vi "波形采集.vi"(2 "rate":dbl=4000.0, 3 "number of samples":i32=1000, 5 "error in":errorcluster) -> ()   [LabVIEW 2010]
doc: "Creates, edits, and runs tasks using NI-DAQmx. Refer to the DAQ Quick Start Guide for information on devices supported by NI-DAQmx.\n\nWhen you place this Express VI on the block diagram, the DAQ Assistant launches to create a new task. After you create a task, you can double-click the DAQ Assistant Express VI in order to edit that task. For continuous measurement or generation, place a loop around the DAQ Assistant Express VI. \n\nFor continuous single-point input or output, the DAQ Assistant Express VI might not provide satisfactory performance. Refer to examples\\DAQmx\\Analog In\\Measure Voltage.llb\\Cont Acq&Graph Voltage-Single Point Optimization.vi for techniques to create higher-performance, single-point I/O applications."
uses:
  <vilib>/DAQmx/read.llb/DAQmx Read (Analog 1D Wfm NChan NSamp).vi
  <vilib>/DAQmx/configure/timing.llb/DAQmx Timing (Sample Clock).vi
  <vilib>/DAQmx/create/channels.llb/DAQmx Create Channel (TEDS-AI-Voltage-Basic).vi
  <vilib>/DAQmx/create/channels.llb/DAQmx Create Channel (AI-Voltage-Basic).vi
  <vilib>/daqmx/miscellaneous.llb/DAQmx Fill In Error Info.vi
panel:
  in  "停止":bool
  out "波形图":waveform(dbl)[](graph)
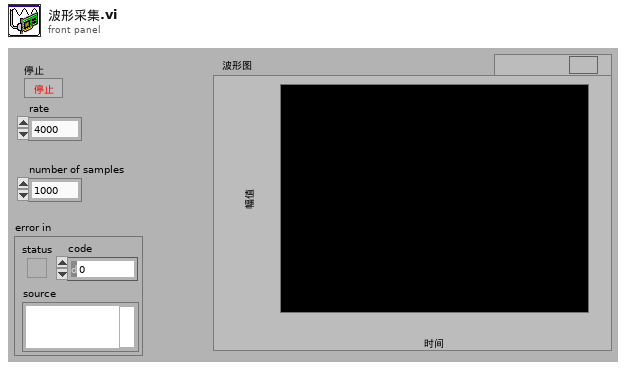
[diagram p1: front panel]
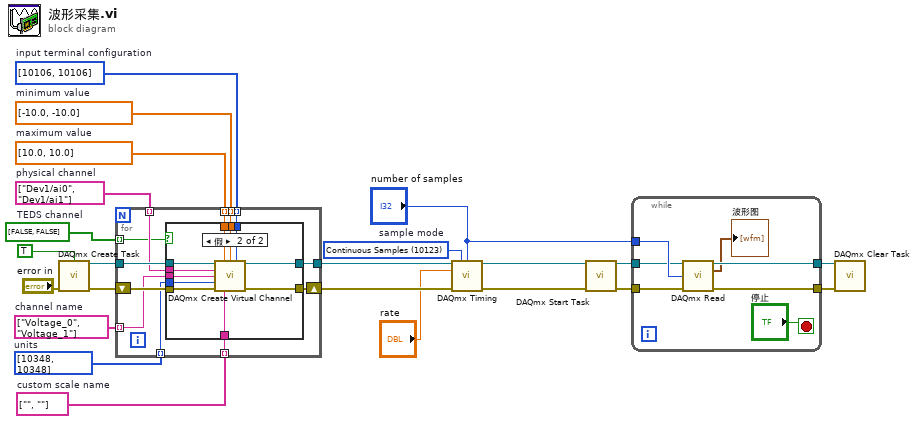
[diagram p0: block diagram]
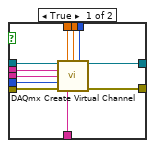
[diagram p2: hidden frame]
diagram:
  w6 = 10123 items=["Finite Samples"=10178, "Continuous Samples"=10123, "Hardware Timed Single Point"=12522]  # sample mode
  w11 = bool[] [FALSE, FALSE]  # TEDS channel
  w12 = string[] ["", ""]  # custom scale name
  w13 = i32[] [10348, 10348] items=["Volts"=10348, "From TEDS"=12516, "From Custom Scale"=10065]  # units
  w14 = string[] ["Voltage_0", "Voltage_1"]  # channel name
  w15 = string[] ["Dev1/ai0", "Dev1/ai1"]  # physical channel
  w16 = dbl[] [10.0, 10.0]  # maximum value
  w17 = dbl[] [-10.0, -10.0]  # minimum value
  w18 = i32[] [10106, 10106] items=["default"=-1, "RSE"=10083, "NRSE"=10078, "Differential"=10106, "Pseudodifferential"=12529]  # input terminal configuration
  n1 = call <vilib>:"DAQmx Create Task.vi"("auto cleanup"=TRUE, "error in"="error in") -> ("task out"=w23:refnum<k21>, "error out"=w22:errorcluster)  [unwired: 12 in]
  n2 = for "For循环" {
    tunnel: w23 -> [w35]
    tunnel: [w33] -> w20
    tunnel: w18 -> [w31] mode=indexing
    tunnel: w17 -> [w30] mode=indexing
    tunnel: w16 -> [w29] mode=indexing
    tunnel: w15 -> [w28] mode=indexing
    tunnel: w14 -> [w27] mode=indexing
    tunnel: w13 -> [w26] mode=indexing
    tunnel: w12 -> [w25] mode=indexing
    shift-right: [w32] -> w19
    shift-left: w22 -> [w34]
    tunnel: w11 -> [w24] mode=indexing
    n3 = case "条件结构" shown="假" w24 {
      tunnel: w35 -> [w46 w57]
      tunnel: w34 -> [w45 w56]
      tunnel: [w44 w55] -> w33
      tunnel: [w43 w54] -> w32
      tunnel: w31 -> [w42 w53]
      tunnel: w30 -> [w41 w52]
      tunnel: w29 -> [w40 w51]
      tunnel: w28 -> [w39 w50]
      tunnel: w27 -> [w38 w49]
      tunnel: w26 -> [w37 w48]
      tunnel: w25 -> [w36 w47]
      frame True {
        n4 = call-poly <vilib>:"DAQmx Create Virtual Channel.vi"("task in"=w46, "maximum value"=w40, "minimum value"=w41, "input terminal configuration"=w42, "physical channels"=w39, "name to assign"=w38, "units"=w37, "error in"=w45, "custom scale name"=w36) -> ("task out"=w44:refnum<k21>, "error out"=w43:errorcluster)  [unwired: 5 in]
      }
      frame False {
        n5 = call-poly <vilib>:"DAQmx Create Virtual Channel.vi"("task in"=w57, "maximum value"=w51, "minimum value"=w52, "input terminal configuration"=w53, "physical channels"=w50, "name to assign"=w49, "units"=w48, "error in"=w56, "custom scale name"=w47) -> ("task out"=w55:refnum<k21>, "error out"=w54:errorcluster)  [unwired: 5 in]
      }
    }
  }
  n6 = call-poly <vilib>:"DAQmx Timing.vi"("task/channels in"=w20, "sample mode"=w6, "samples per channel"="number of samples", "rate"="rate", "error in"=w19) -> ("task out"=w10:refnum<k21>, "error out"=w9:errorcluster)  [unwired: 9 in]
  n7 = call <vilib>:"DAQmx Start Task.vi"("task/channels in"=w10, "error in"=w9) -> ("task out"=w5:refnum<k21>, "error out"=w4:errorcluster)  [unwired: 12 in]
  n8 = while {
    tunnel: "number of samples" -> [w64]
    tunnel: w5 -> [w63]
    tunnel: w4 -> [w62]
    tunnel: [w61] -> w1
    tunnel: [w60] -> w2
    stop <- "停止" stop-if-true
    n9 = call-poly <vilib>:"DAQmx Read.vi"("task/channels in"=w63, "number of samples per channel"=w64, "error in"=w62) -> ("task out"=w60:refnum<k21>, "data"=→"波形图":waveform(dbl)[], "error out"=w61:errorcluster)  [unwired: 10 in]
  }
  n10 = call <vilib>:"DAQmx Clear Task.vi"("task in"=w2, "error in"=w1) -> ()  [unwired: 13 in, 1 out]
